vi "UE_LV2.vi"   [LabVIEW 2021]
doc: "Polymorphic VI to take many of input data type"
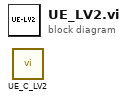
[diagram p0: block diagram]
diagram:
  n1 = call "UE_C_LV2.vi"() -> ()  [unwired: 14 in, 2 out]
